vi "Print VS Debug String.vi"(8 "error in (no error)":errorcluster, 10 "Append Error (T)":bool=TRUE, 11 "String":string) -> (0 "error out":errorcluster)   [LabVIEW 2020, in "FPGA Addon Engine.lvlib"]
uses:
  FPGA Addon Engine.lvlib
  <vilib>/NI VeriStand/Custom Device Tools/Custom Device Utility Library/Custom Device Utility Library.lvlib
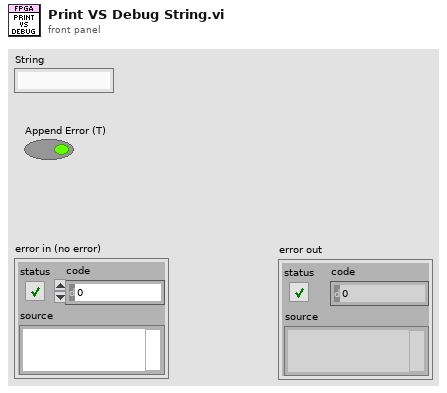
[diagram p1: front panel]
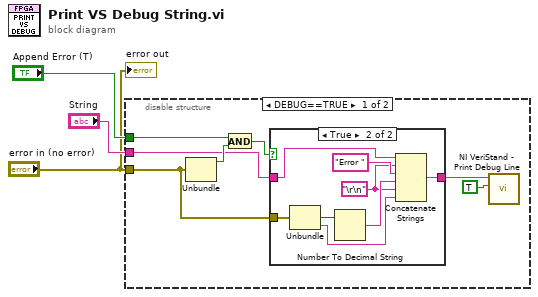
[diagram p0: block diagram]
diagram:
  n1 = disable-structure shown="DEBUG==TRUE" {
    disable-tunnel: "Append Error (T)" -> [w9 _]
    disable-tunnel: "String" -> [w7 _]
    disable-tunnel: "error in (no error)" -> [w6 _]
    frame condition #0 (active) {
      n2 = Unbundle(w6) -> ("status"=w8:bool)  [unwired: 2 out]
      n3 = And(x=w9, y=w8) -> (x .and. y?=w10:bool)
      n4 = case shown="True" w10 {
        tunnel: w7 -> [w11 w19]
        tunnel: w6 -> [_ w18]
        tunnel: [w11 w12] -> w4
        frame False {
        }
        frame True {
          w14 = "\r\n" ("string")
          n5 = Unbundle(w18) -> ("code"=w16:i32, "source"=w13:string)  [unwired: 1 out]
          n6 = Number To Decimal String(number=w16) -> (decimal integer string=w15:string)  [unwired: 1 in]
          n7 = Concatenate Strings(w19, w14, "Error " ("string"), w15, w14, w13) -> (w12:string)
        }
      }
      n8 = call <vilib>:"NI VeriStand - Print Debug Line.vi"("Add to log file? (F)"=TRUE, "Message"=w4) -> ()  [unwired: 9 in, 1 out]
    }
    frame condition #1 {
    }
  }
  "error out" <- "error in (no error)"
